vi "RPC Method Measurement_v1_MeasurementService_GetMetadata.vi"(8 "error in (no error)":errorcluster, 10 "Request Data":T7, 11 "gRPC Client in":refnum<class "Measurement_lv_client.lvclass">) -> (0 "error out":errorcluster, 2 "Response Data":T1, 3 "gRPC Client out":refnum<class "Measurement_lv_client.lvclass">)   [LabVIEW 2020, in "Measurement_lv_client.lvlib" / "Measurement_lv_client.lvclass"]
uses:
  Measurement_lv_client.lvclass
  RPC Messages/Measurement_v1_GetMetadataRequest/Measurement_v1_GetMetadataRequest_Data.ctl
  RPC Messages/Measurement_v1_GetMetadataResponse/Measurement_v1_GetMetadataResponse_Data.ctl
  RPC Messages/Measurement_v1_MeasurementDetails/Measurement_v1_MeasurementDetails_Data.ctl
  RPC Messages/Measurement_v1_MeasurementParameters/Measurement_v1_MeasurementParameters_Data.ctl
  RPC Messages/Measurement_v1_ConfigurationParameter/Measurement_v1_ConfigurationParameter_Data.ctl
  RPC Messages/Measurement_v1_OutputParameter/Measurement_v1_OutputParameter_Data.ctl
  RPC Messages/Measurement_v1_UserInterfaceDetails/Measurement_v1_UserInterfaceDetails_Data.ctl
  Measurement_lv_client.lvclass/Measurement_lv_client.ctl
  fa22ca14-33b2-4bc3-8699-3f27c9b27c9c.vi
  <vilib>/gRPC/LabVIEW gRPC Library/Server API/Server/Get Server DLL Path.vi
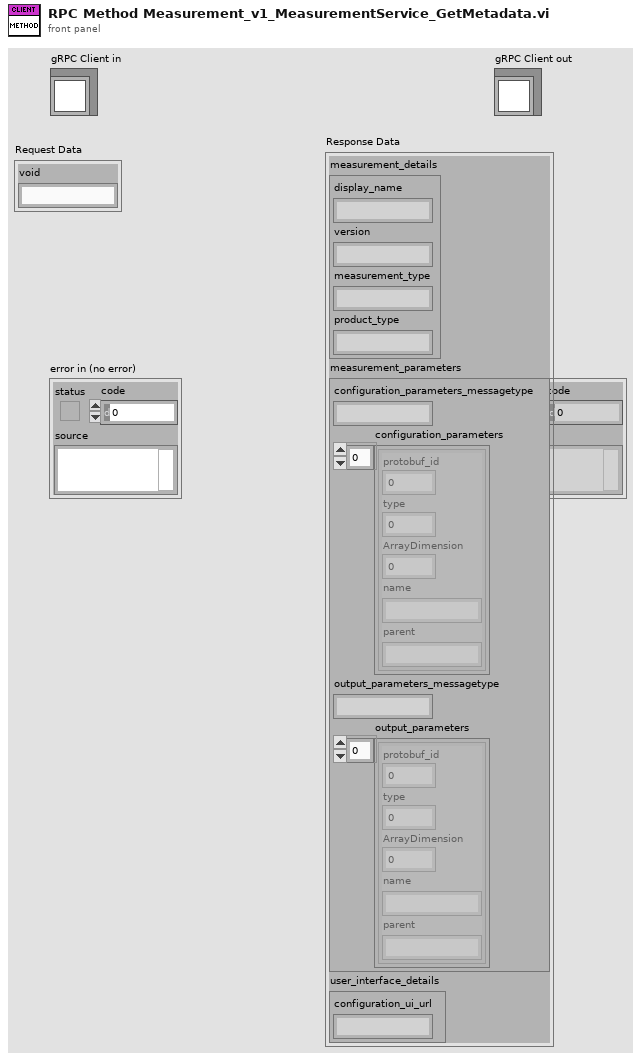
[diagram p1: front panel]
types:
  T1 = typedef "Measurement_lv_client.lvlib/Measurement_lv_client.lvclass/Measurement_v1_GetMetadataResponse_Data.ctl" = cluster{"measurement_details":T2, "measurement_parameters":T3, "user_interface_details":T6}
  T2 = typedef "Measurement_lv_client.lvlib/Measurement_lv_client.lvclass/Measurement_v1_MeasurementDetails_Data.ctl" = cluster{"display_name":string, "version":string, "measurement_type":string, "product_type":string}
  T3 = typedef "Measurement_lv_client.lvlib/Measurement_lv_client.lvclass/Measurement_v1_MeasurementParameters_Data.ctl" = cluster{"configuration_parameters_messagetype":string, "configuration_parameters":T4[], "output_parameters_messagetype":string, "output_parameters":T5[]}
  T4 = typedef "Measurement_lv_client.lvlib/Measurement_lv_client.lvclass/Measurement_v1_ConfigurationParameter_Data.ctl" = cluster{"protobuf_id":i32, "type":i32, "ArrayDimension":i32, "name":string, "parent":string}
  T5 = typedef "Measurement_lv_client.lvlib/Measurement_lv_client.lvclass/Measurement_v1_OutputParameter_Data.ctl" = cluster{"protobuf_id":i32, "type":i32, "ArrayDimension":i32, "name":string, "parent":string}
  T6 = typedef "Measurement_lv_client.lvlib/Measurement_lv_client.lvclass/Measurement_v1_UserInterfaceDetails_Data.ctl" = cluster{"configuration_ui_url":string}
  T7 = typedef "Measurement_lv_client.lvlib/Measurement_lv_client.lvclass/Measurement_v1_GetMetadataRequest_Data.ctl" = cluster{"void":string}
  T8 = typedef "gprc-lvsupport-release.lvlib/grpcId.ctl" = u64
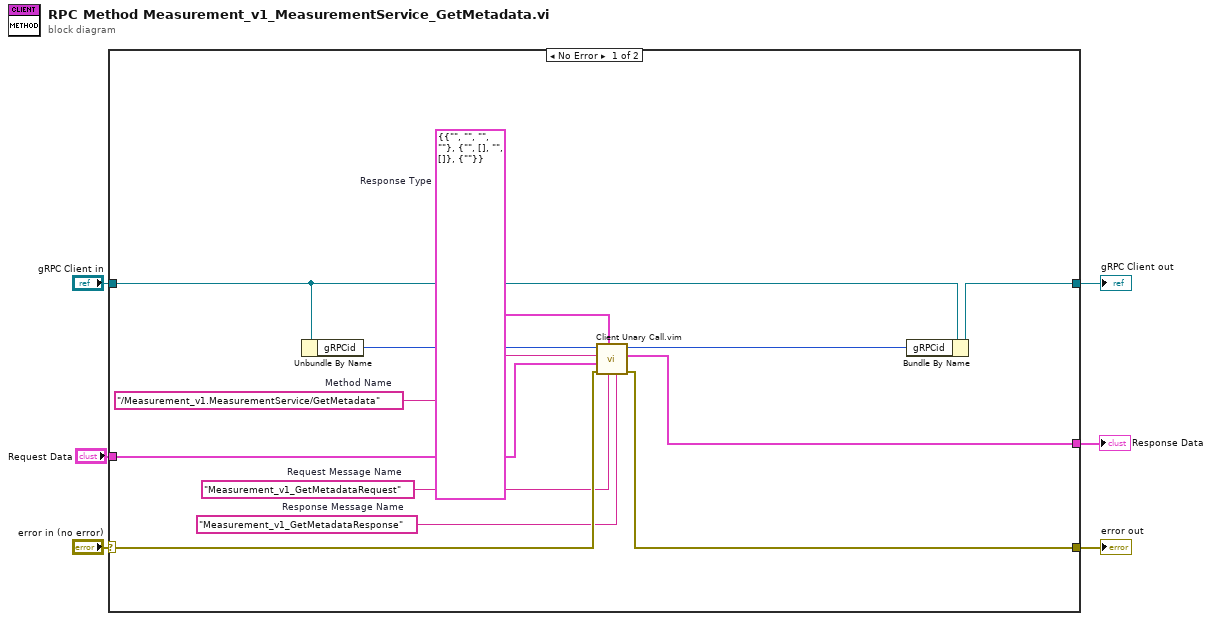
[diagram p0: block diagram]
diagram:
  n1 = case shown="No Error" "error in (no error)" {
    selector: "error in (no error)" -> [w14 w20]
    tunnel: [w13 w20] -> w5
    tunnel: [w15 w19] -> w3
    tunnel: "gRPC Client in" -> [w17 w19]
    tunnel: "Request Data" -> [w11 _]
    tunnel: [w10 _] -> w1
    frame No Error {
      w7 = "Measurement_v1_GetMetadataResponse"  # Response Message Name
      w8 = "Measurement_v1_GetMetadataRequest"  # Request Message Name
      w9 = T1 {"measurement_details"={"display_name"="", "version"="", "measurement_type"="", "product_type"=""}, "measurement_parameters"={"configuration_parameters_messagetype"="", "configuration_parameters"=[], "output_parameters_messagetype"="", "output_parameters"=[]}, "user_interface_details"={"configuration_ui_url"=""}}  # Response Type
      w12 = "/Measurement_v1.MeasurementService/GetMetadata"  # Method Name
      n2 = Unbundle By Name(w17) -> ("gRPCid"=w18:T8)
      n3 = call "Client Unary Call.vim"("Response Message Name"=w7, "Request Message Name"=w8, "Response Type"=w9, "error in (no error)"=w14, "Request Data"=w11, "Method Name"=w12, "Client Ref"=w18) -> ("error out"=w13:errorcluster, "Response Data"=w10:T1, "Client Ref Out"=w16:u64)  [unwired: 2 in]
      n4 = Bundle By Name(cluster=w17, "gRPCid"=w16) -> (w15:refnum<class "Measurement_lv_client.lvclass">)
    }
    frame Error {
    }
  }
  "error out" <- w5
  "gRPC Client out" <- w3
  "Response Data" <- w1
